vi "Resample image by X.vi"(8 "error in (no error)":errorcluster, 9 "Resampled Image Name":string="First", 10 "X Resolution":i32=500, 11 "Refnum in":T1) -> (3 "Refnum out":T1)   [LabVIEW 2020]
uses:
  <vilib>/vision/Image Controls.llb/IMAQ Image.ctl
  <vilib>/vision/NI_Vision_Development_Module.lvlib
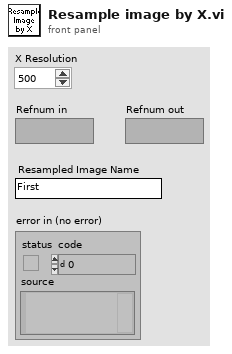
[diagram p1: front panel]
types:
  T1 = typedef "IMAQ Image.ctl" = refnum<image>
  T2 = typedef "Image Type" = u32
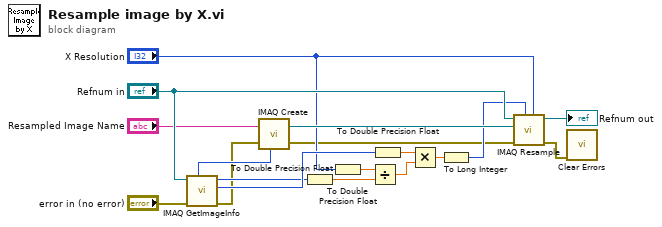
[diagram p0: block diagram]
diagram:
  n1 = call "IMAQ GetImageInfo"("error in (no error)"="error in (no error)", "Image"="Refnum in") -> ("error out"=w4:errorcluster, "Y Resolution"=w8:i32, "X Resolution"=w7:i32, "Image Type"=w17:T2)  [unwired: 2 in, 4 out]
  n2 = call "IMAQ Create"("Image Name"="Resampled Image Name", "Image Type"=w17, "error in (no error)"=w4) -> ("New Image"=w18:T1, "error out"=w3:errorcluster)  [unwired: 2 in]
  n3 = To Double Precision Float(number=w7) -> (double precision float=w10:dbl)
  n4 = To Double Precision Float(number="X Resolution") -> (double precision float=w5:dbl)
  n5 = Divide(x=w5, y=w10) -> (x/y=w13:dbl)
  n6 = To Double Precision Float(number=w8) -> (double precision float=w11:dbl)
  n7 = Multiply(x=w11, y=w13) -> (x*y=w12:dbl)
  n8 = To Long Integer(number=w12) -> (32bit integer=w9:i32)
  n9 = call "IMAQ Resample"("X Resolution"="X Resolution", "Y Resolution"=w9, "error in (no error)"=w3, "Image Dst"=w18, "Image Src"="Refnum in") -> ("error out"=w2:errorcluster, "Image Dst Out"=→"Refnum out":T1)  [unwired: 5 in]
  n10 = call <vilib>:"Clear Errors.vi"("error in (no error)"=w2) -> ()  [unwired: 5 in, 2 out]
